vi "Partial Cluster With Array Of Digital Data.vi"(8 "LV Control Name Paths":string[](array[string]), 9 "TS Variable Name Paths":string[](array[string]), 10 "Sequence Context":refnum<k7>, 11 "Cluster":cluster{"Numeric":dbl, "Array":digitaldata[]}={"Numeric"=0.0, "Array"=[{"transitions"=[], "data"=[]}]}) -> (0 "error out":errorcluster, 1 "Report Text":string, 2 "PASS/FAIL Flag":bool, 3 "Cluster 2":cluster{"Numeric":dbl, "Array":digitaldata[]})   [LabVIEW 2013]
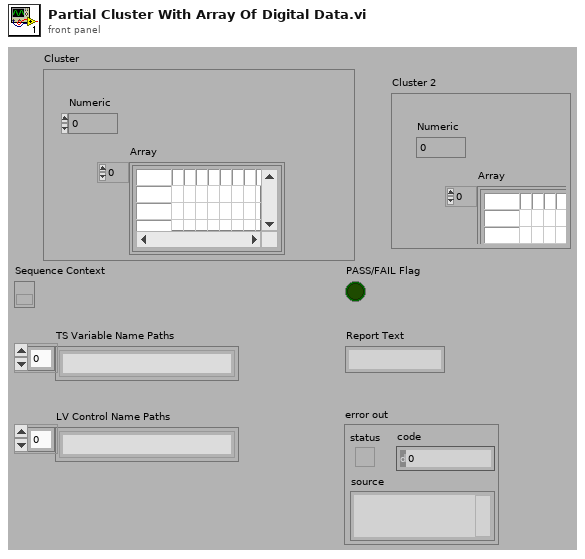
[diagram p1: front panel]
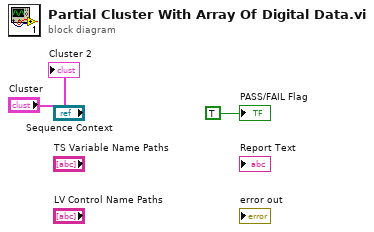
[diagram p0: block diagram]
diagram:
  "PASS/FAIL Flag" <- TRUE ("PASS/FAIL Flag")
  "Cluster 2" <- "Cluster"
